vi "Get_Intensity_Value_For_Thresholding-2.vi"(4 "[IN] Index for \nthresholding":i8, 5 "error IN":errorcluster, 6 "[IN] Binarization Set\ntings (Both Channels)":cluster{"MinBin2":sgl, "MaxBin2":sgl}[](array[cluster]), 7 "[IN] 1 or 2 channel":u8, 8 "[IN] Index of starting \npoint for thresholding":i32) -> (0 "error OUT":errorcluster, 1 "[OUT] Binarization Set\ntings (Both Channels)":cluster{"MinBin2":sgl, "MaxBin2":sgl}[](array[cluster]), 2 "[OUT] For Operator \nBinarization Values":cluster{"MinBin2":sgl, "MaxBin2":sgl})   [LabVIEW 2017]
doc: "SubVI saves used for thresholding limits (255 - commonly highest value, user defines only 1 value for threshold)"
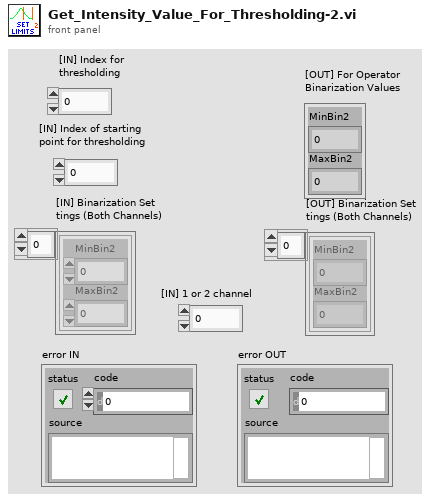
[diagram p1: front panel]
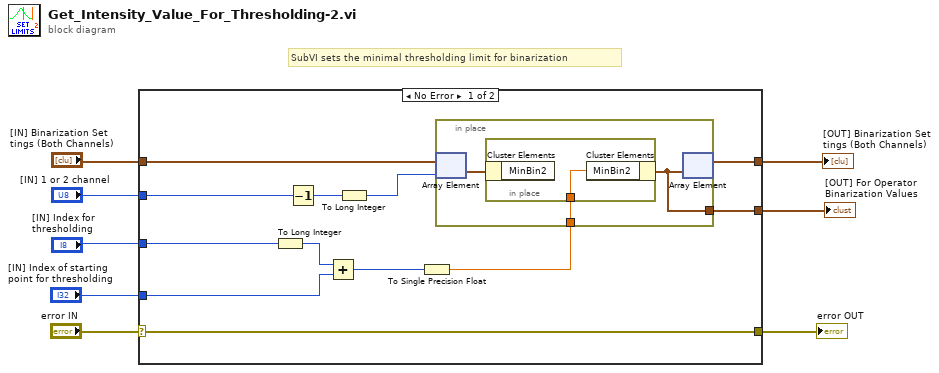
[diagram p0: block diagram]
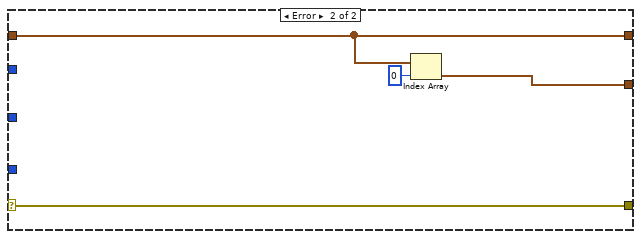
[diagram p2: hidden frame]
diagram:
  # "SubVI sets the minimal thresholding limit for binarization"
  n1 = case shown="No Error" "error IN" {
    selector: "error IN" -> [w18 w28]
    tunnel: [w18 w28] -> w7
    tunnel: [w14 w27] -> w5
    tunnel: "[IN] Binarization Set\ntings (Both Channels)" -> [w13 w27]
    tunnel: [w12 w25] -> w4
    tunnel: "[IN] Index for \nthresholding" -> [w11 _]
    tunnel: "[IN] Index of starting \npoint for thresholding" -> [w10 _]
    tunnel: "[IN] 1 or 2 channel" -> [w9 _]
    frame No Error {
      n2 = To Long Integer(number=w11) -> (32bit integer=w19:i32)
      n3 = Decrement(x=w9) -> (x-1=w17:u8)
      n4 = Add(x=w19, y=w10) -> (x+y=w20:i32)
      n5 = To Long Integer(number=w17) -> (32bit integer=w16:i32)
      n6 = To Single Precision Float(number=w20) -> (single precision float=w15:sgl)
      n7 = in-place {
        in-place-border: w15 -> [w22]
        in-place-border: [w21] -> w12
        n8 = in-place-array #1(w13, w16) -> (w23:cluster{"MinBin2":sgl, "MaxBin2":sgl})
        n9 = in-place {
          in-place-border: w22 -> [w24]
          n10 = in-place-cluster #2(w23) -> ()  [unwired: 1 out]
          n11 = in-place-cluster #2("MinBin2"=w24) -> (w21:cluster{"MinBin2":sgl, "MaxBin2":sgl})
        }
        n12 = in-place-array #1(w21) -> (w14:cluster{"MinBin2":sgl, "MaxBin2":sgl}[])  [unwired: 1 out]
      }
    }
    frame Error {
      n13 = Index Array(array=w27, index=0) -> (element=w25:cluster{"MinBin2":sgl, "MaxBin2":sgl})
    }
  }
  "error OUT" <- w7
  "[OUT] Binarization Set\ntings (Both Channels)" <- w5
  "[OUT] For Operator \nBinarization Values" <- w4
